vi "Search 1D Array Function.vi"() -> ()   [LabVIEW 2014]
panel:
  out "元素索引":i32
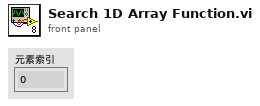
[diagram p1: front panel]
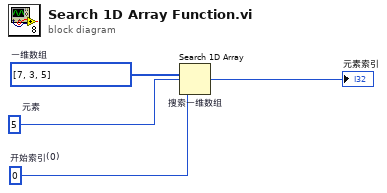
[diagram p0: block diagram]
diagram:
  w3 = 0  # 开始索引(0)
  w2 = 5  # 元素
  w4 = i32[] [7, 3, 5]  # 一维数组
  n1 = Search 1D Array "搜索一维数组"(1D array=w4, element=w2, start index (0)=w3) -> (index of element=→"元素索引":i32)
